vi "报警更新.vi"(9 "Message Data":variant, 10 "state":string="报警更新") -> ()   [LabVIEW 2015]
uses:
  <userlib>/QMH/Message Queue/Support/Enqueue Message (Single).vi
  <userlib>/QMH/Message Queue/Message Queue.lvlib
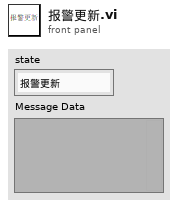
[diagram p1: front panel]
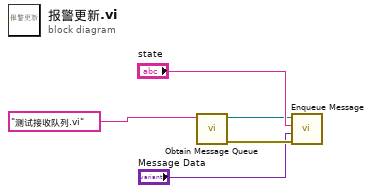
[diagram p0: block diagram]
diagram:
  n1 = call <userlib>:"Obtain Message Queue.vi"("name (unnamed)"="测试接收队列.vi" ("name")) -> ("error out"=w4:errorcluster, "Message Queue"=w3:refnum<queue>)  [unwired: 9 in]
  n2 = call-poly <userlib>:"Enqueue Message.vi"("error in (no error)"=w4, "Message Data"="Message Data", "Message"="state", "Message Queue"=w3) -> ()  [unwired: 6 in, 2 out]
